vi "Run Service.vi"(7 "measurement":refnum<class "Measurement Plugin Service.lvclass">, 8 "error in":errorcluster, 11 "measurementlink server user settings":T1) -> (0 "error out":errorcluster)   [LabVIEW 2020, in "Measurement Plugin Measurement Server.lvlib"]
uses:
  Measurement Plugin Measurement Server.lvlib
  <vilib>/gRPC/LabVIEW gRPC Servicer/Servicer/Servicer.lvclass
  Measurement Plugin Discovery Client/Measurement Plugin Discovery Client.lvlib
  IMeasurement Service/IMeasurement Service.lvclass
  Measurement Plugin Service/Measurement Plugin Service.lvclass
  Measurement Plugin Discovery V1/Measurement Plugin Discovery V1.lvlib
  Helpers/TypeDefs/Measurement Server User Settings.ctl
  Helpers/TypeDefs/Stop Server User Event.ctl
  Helpers/TypeDefs/Measurement Service Version.ctl
panel:
  out "Display Name":string
  out "Listening Port":i32
  in  "Stop":bool
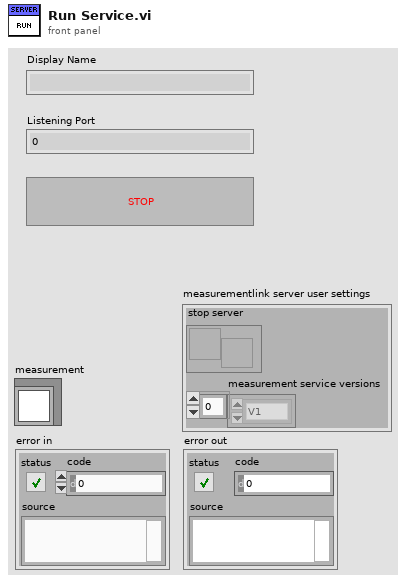
[diagram p1: front panel]
types:
  T1 = typedef "Measurement Plugin Measurement Server.lvlib/Measurement Server User Settings.ctl" = cluster{"stop server":T2, "measurement service versions":T3[]}
  T2 = typedef "Measurement Plugin Measurement Server.lvlib/Stop Server User Event.ctl" = refnum<user-event>
  T3 = typedef "Measurement Plugin Measurement Server.lvlib/Measurement Service Version.ctl" = enum16{"V1", "V2"}
  T4 = enum32{"Invalid", "Standard", "Closed", "Hidden", "Minimized", "Maximized"}
  T5 = typedef "Measurement Plugin Measurement Server.lvlib/Measurement Details.ctl" = cluster{"display name":string, "version":string}
  T6 = typedef "grpc-lvsupport-release.lvlib/grpcId.ctl" = u64
  T7 = typedef "Measurement Plugin Discovery Client.lvlib/ni_measurementlink_discovery_v1_RegisterServiceResponse.ctl" = cluster{"registration_id":string}
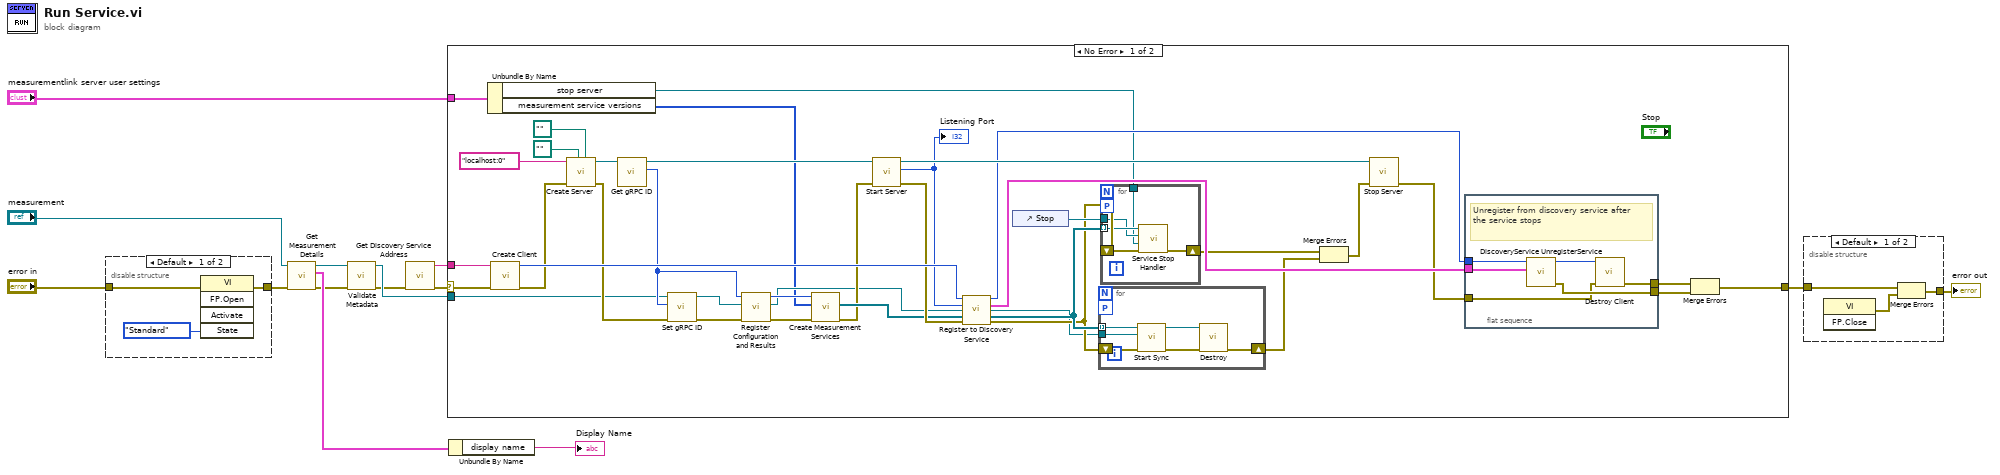
[diagram p0: block diagram]
diagram:
  n1 = disable-structure shown="Default" {
    disable-tunnel: [w16 w18] -> w8
    disable-tunnel: "error in" -> [w15 w18]
    frame condition #0 (active) {
      n2 = invoke class="VI" method="FP.Open"(error in=w15, "State"=T4."Standard") -> (error out=w16:errorcluster)  [unwired: 3 in, 4 out]
    }
    frame condition #1 {
    }
  }
  n3 = call-dynamic "Get Measurement Details.vi"("error in"=w8, "measurement plugin service in"="measurement") -> ("error out"=w2:errorcluster, "measurement details"=w10:T5, "measurement plugin service out"=w4:refnum<class "Measurement Plugin Service.lvclass">)  [unwired: 5 in, 2 out]
  n4 = call "Validate Metadata.vi"("error in"=w2, "measurement plugin service in"=w4) -> ("error out"=w1:errorcluster, "measurement plugin service out"=w3:refnum<class "Measurement Plugin Service.lvclass">)  [unwired: 8 in]
  n5 = call "Get Discovery Service Address.vi"("error in"=w1) -> ("error out"=w14:errorcluster, "address"=w13:string)  [unwired: 9 in]
  n6 = case shown="No Error" w14 {
    selector: w14 -> [w22 w74]
    tunnel: [w56 w74] -> w6
    tunnel: w3 -> [w21 _]
    tunnel: w13 -> [w55 _]
    tunnel: "measurementlink server user settings" -> [w20 _]
    frame No Error {
      n7 = Unbundle By Name(w20) -> ("stop server"=w23:T2, "measurement service versions"=w19:T3[])
      n8 = call "Create Client.vi"("error in"=w22, "address"=w55) -> ("error out"=w44:errorcluster, "gRPC ID Out"=w48:T6)  [unwired: 8 in]
      n9 = call <vilib>:"Create Server.vi"("Server Key File (.key)"=path "", "Server Certificate File (.crt)"=path "", "error in"=w44, "Server Address"="localhost:0") -> ("error out"=w33:errorcluster, "gRPC Server out"=w50:refnum<class "Servicer.lvclass">)  [unwired: 6 in]
      n10 = call <vilib>:"Get gRPC ID.vi"("OOP Server in"=w50) -> ("gRPC ID"=w31:T6, "OOP Server out"=w49:refnum<class "Servicer.lvclass">)  [unwired: 9 in]
      n11 = call "Set gRPC ID.vi"("error in"=w33, "gRPC ID"=w31, "measurement plugin service in"=w21) -> ("error out"=w32:errorcluster, "measurement plugin service out"=w30:refnum<class "Measurement Plugin Service.lvclass">)  [unwired: 7 in]
      n12 = call "Register Configuration and Results.vi"("error in"=w32, "measurement plugin service in"=w30, "gRPC ID in"=w31) -> ("error out"=w29:errorcluster, "measurement plugin service out"=w25:refnum<class "Measurement Plugin Service.lvclass">, "gRPC ID out"=w28:T6)  [unwired: 6 in]
      n13 = call "Create Measurement Services.vi"("error in"=w29, "measurement service versions"=w19, "gRPC ID in"=w28) -> ("error out"=w26:errorcluster, "measurement service array out"=w27:refnum<class "IMeasurement Service.lvclass">[])  [unwired: 6 in, 1 out]
      n14 = call <vilib>:"Start Server.vi"("error in"=w26, "gRPC Server in"=w49) -> ("error out"=w41:errorcluster, "Listening Port"=w45:i32, "gRPC Server out"=w54:refnum<class "Servicer.lvclass">)  [unwired: 7 in]
      "Listening Port" <- w45
      n15 = call "Register to Discovery Service.vi"("gRPC ID in"=w48, "port number"=w45, "measurement plugin service in"=w25, "measurement service in"=w27, "error in"=w41) -> ("gRPC ID out"=w47:T6, "response data"=w46:T7, "measurement plugin service out"=w24:refnum<class "Measurement Plugin Service.lvclass">, "measurement service out"=w37:refnum<class "IMeasurement Service.lvclass">[], "error out"=w36:errorcluster)  [unwired: 6 in]
      n16 = control-ref of="Stop"() -> (w38:refnum<vi>)
      n17 = for {
        workers-P: _ -> [_]
        tunnel: w37 -> [w62] mode=indexing
        tunnel: w24 -> [w61]
        shift-right: [w58] -> w35
        shift-left: w36 -> [w60]
        n18 = call-dynamic "Start Sync.vi"("error in"=w60, "measurement plugin service in"=w61, "measurement service in"=w62) -> ("error out"=w59:errorcluster, "measurement service out"=w57:refnum<class "IMeasurement Service.lvclass">)  [unwired: 7 in]
        n19 = call-dynamic "Destroy.vi"("error in"=w59, "measurement service in"=w57) -> ("error out"=w58:errorcluster)  [unwired: 9 in]
      }
      n20 = for {
        workers-P: _ -> [_]
        tunnel: w37 -> [w67] mode=indexing
        tunnel: w38 -> [w66]
        shift-right: [w64] -> w34
        shift-left: w36 -> [w65]
        tunnel: w23 -> [w63]
        n21 = call-dynamic "Service Stop Handler.vi"("error in"=w65, "stop server user event"=w63, "stop button ref"=w66, "measurement service in"=w67) -> ("error out"=w64:errorcluster)  [unwired: 6 in, 1 out]
      }
      n22 = Merge Errors(w34, w35) -> (w43:errorcluster)
      n23 = call <vilib>:"Stop Server.vi"("error in"=w43, "gRPC Server in"=w54) -> ("error out"=w42:errorcluster)  [unwired: 9 in]
      n24 = flat-sequence {
        tunnel: w47 -> [w73]
        tunnel: w46 -> [w72]
        tunnel: [w71] -> w40
        tunnel: w42 -> [w68]
        tunnel: [w69] -> w39
        frame #0 {
          # "Unregister from discovery service after the service stops"
          n25 = call "DiscoveryService UnregisterService.vi"("Request Data"=w72, "gRPC ID"=w73) -> ("error out"=w69:errorcluster, "gRPC ID out"=w70:T6)  [unwired: 7 in, 1 out]
          n26 = call "Destroy Client.vi"("error in"=w68, "gRPC ID"=w70) -> ("error out"=w71:errorcluster)  [unwired: 9 in]
        }
      }
      n27 = Merge Errors(w40, w39) -> (w56:errorcluster)
    }
    frame Error {
    }
  }
  n28 = Unbundle By Name(w10) -> ("display name"=→"Display Name":string)
  n29 = disable-structure shown="Default" {
    disable-tunnel: w6 -> [w77 w78]
    disable-tunnel: [w75 w78] -> w5
    frame condition #0 (active) {
      n30 = invoke class="VI" method="FP.Close"() -> (error out=w76:errorcluster)  [unwired: 3 in, 2 out]
      n31 = Merge Errors(w77, w76) -> (w75:errorcluster)
    }
    frame condition #1 {
    }
  }
  "error out" <- w5
